vi "oauth2_authorize_code.vi"(8 "error in (no error)":errorcluster, 10 "redirect_uri":string, 11 "client_id":string) -> (0 "error out":errorcluster, 3 "auth_url":string)   [LabVIEW 2015, in "lv-dropbox.lvlib"]
uses:
  lv-dropbox.lvlib
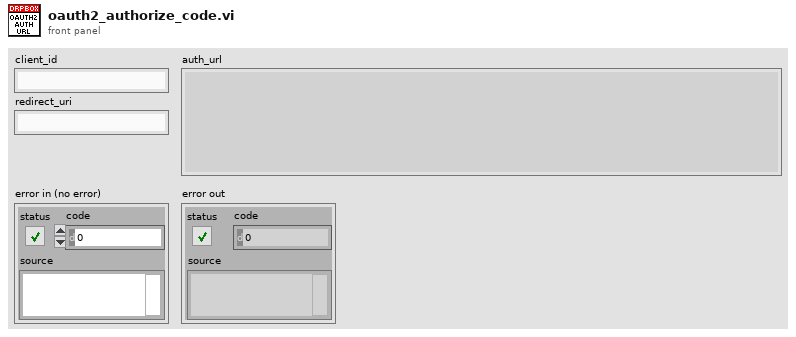
[diagram p1: front panel]
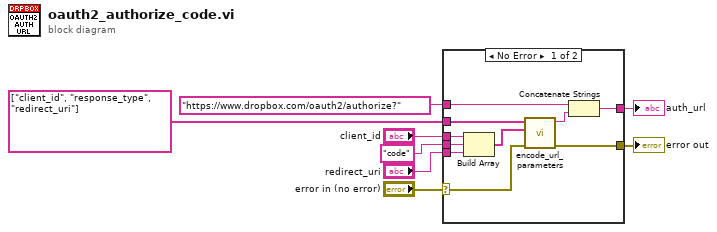
[diagram p0: block diagram]
diagram:
  n1 = case shown="No Error" "error in (no error)" {
    selector: "error in (no error)" -> [w16 w19]
    tunnel: [w17 w19] -> w6
    tunnel: "https://www.dropbox.com/oauth2/authorize?" ("url") -> [w9 _]
    tunnel: "client_id" -> [w13 _]
    tunnel: [w18 _] -> w4
    tunnel: string[] ["client_id", "response_type", "redirect_uri"] -> [w14 _]
    tunnel: "code" -> [w11 _]
    tunnel: "redirect_uri" -> [w10 _]
    frame No Error {
      n2 = Build Array(w13, w11, w10) -> (w12:string[])
      n3 = call "encode_url_parameters.vi"("error in (no error)"=w16, "value []"=w12, "key []"=w14) -> ("error out"=w17:errorcluster, "url_encoded_string"=w15:string)  [unwired: 7 in]
      n4 = Concatenate Strings(w9, w15) -> (w18:string)
    }
    frame Error {
    }
  }
  "error out" <- w6
  "auth_url" <- w4
